vi "VisualizeNHRRGS.vi"() -> ()   [LabVIEW 2018, in "Visualization.lvlib" / "VisualizeAcPwr.lvclass"]
doc: "This VI listens for any measurement data associated with the provided PluginName and displays it to the user for analysis. The display is only suitable for data coming from the NHR Regenerative Grid Simulator Plugin."
uses:
  VisualizeAcPwr.lvclass
  AcPwr/AcPwrShared/clMeasurmentData.ctl
  <vilib>/event_ctls.llb/usereventprio.ctl
  VisualizeBase/VisualizeBase_class/Requests/VisUserEventType.ctl
  <vilib>/Utility/error.llb/Error Cluster From Error Code.vi
  <vilib>/ErrorRing/Error Ring.xnode
  VisualizeBase/VisualizeBase_class/VisualizeBase.lvclass
  <userlib>/NIST/NISTErrorLib/NISTErrorLib.lvlib
  AcPwr/AcPwrShared/AcPwrShared.lvlib
panel:
  out "NHRRGS":waveform(dbl)[](graph)=[{"t0"=timestamp(3657200531.6397257 s since 1904-01-01), "dt"=1.0, "Y"=[46.19]}, {"t0"=timestamp(3657200531.6397257 s since 1904-01-01), "dt"=1.0, "Y"=[2.0]}, {"t0"=timestamp(3657200531.6397257 s since 1904-01-01), "dt"=1.0, "Y"=[60.0]}]
  out "Status Byte Register":T1(array[cluster])
  out "Incorrect DataType?":bool
  in  "PluginName":string="AcPwr.NHRRGS0"
  in  "PlotYAxis":u32[](array[numeric])=[0, 1, 0] max=1
  out "ErrorArray":errorcluster[](array[cluster])
  in  "btnStop":bool
  in  "btnReset":bool
  in  "btnClear":bool
  # "0=Left Axis and 1=Right Axis"
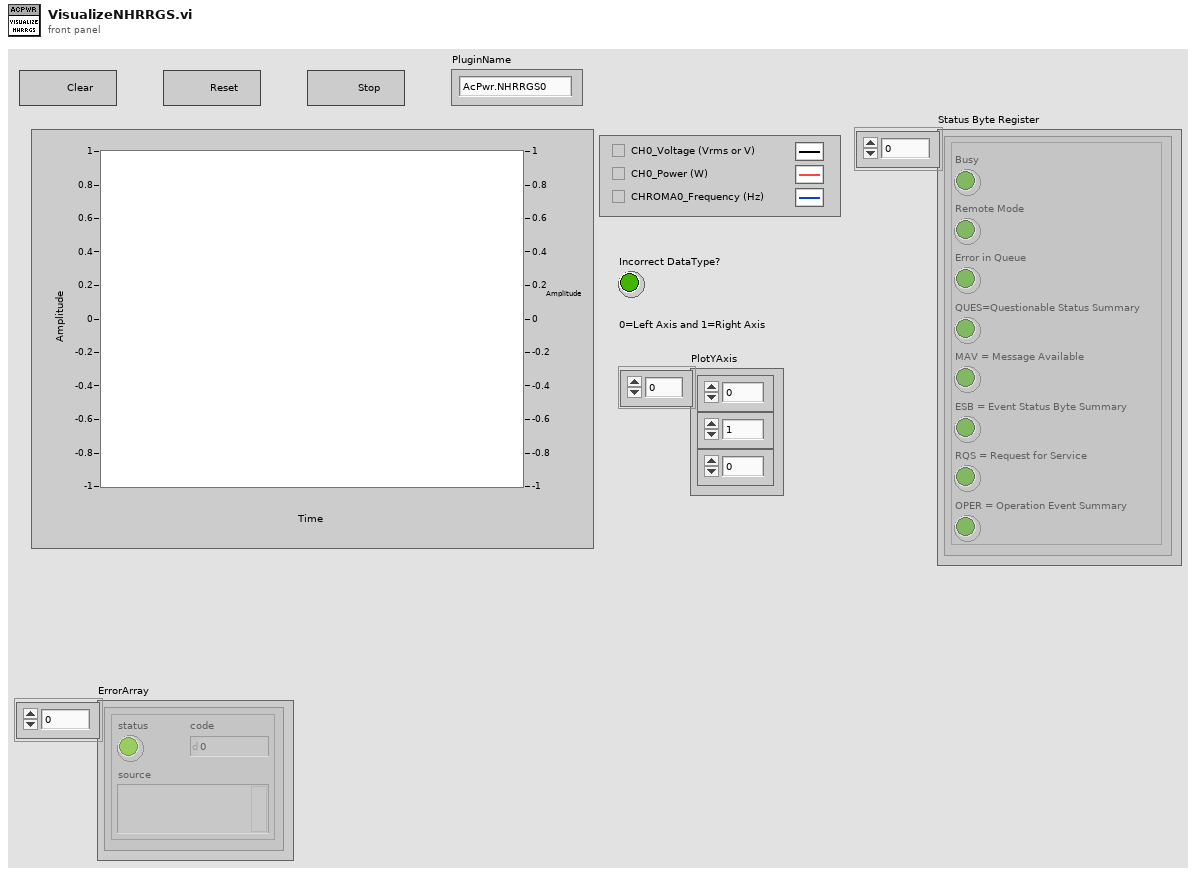
[diagram p1: front panel]
types:
  T1 = cluster{"Busy":bool, "Remote Mode":bool, "Error in Queue":bool, "QUES=Questionable Status Summary":bool, "MAV = Message Available":bool, "ESB = Event Status Byte Summary":bool, "RQS = Request for Service":bool, "OPER = Operation Event Summary":bool}[]
  T2 = typedef "Visualization.lvlib/VisualizeBase.lvclass/VisRequestEvents.ctl" = cluster{"StopRequest":refnum<user-event>, "ResetRequest":refnum<user-event>, "FP Pop In or Out":refnum<user-event>}
  T3 = typedef "AcPwrShared.lvlib/AcPwrBroadcastEvents.ctl" = cluster{"DidInit":refnum<user-event>, "StatusUpdate":refnum<user-event>, "ErrorReport":refnum<user-event>, "DidStop":refnum<user-event>, "PathToINI":refnum<user-event>, "Measurements":refnum<user-event>, "LoadConfigFile":refnum<user-event>, "GetSettings":refnum<user-event>, "SetSettings":refnum<user-event>, "GetType&ID":refnum<user-event>, "GotSettings":refnum<user-event>}
  T4 = typedef "AcPwrShared.lvlib/clMeasurmentData.ctl" = cluster{"MeasName":string, "XML Data":string, "WaveformData":waveform(dbl)[]}
  T5 = typedef "Visualization.lvlib/VisualizeBase.lvclass/VisUserEventType.ctl" = cluster{"BusIndex":i8, "Data":variant}
  T6 = typedef "usereventprio.ctl" = enum32{"high priority", "normal priority"}
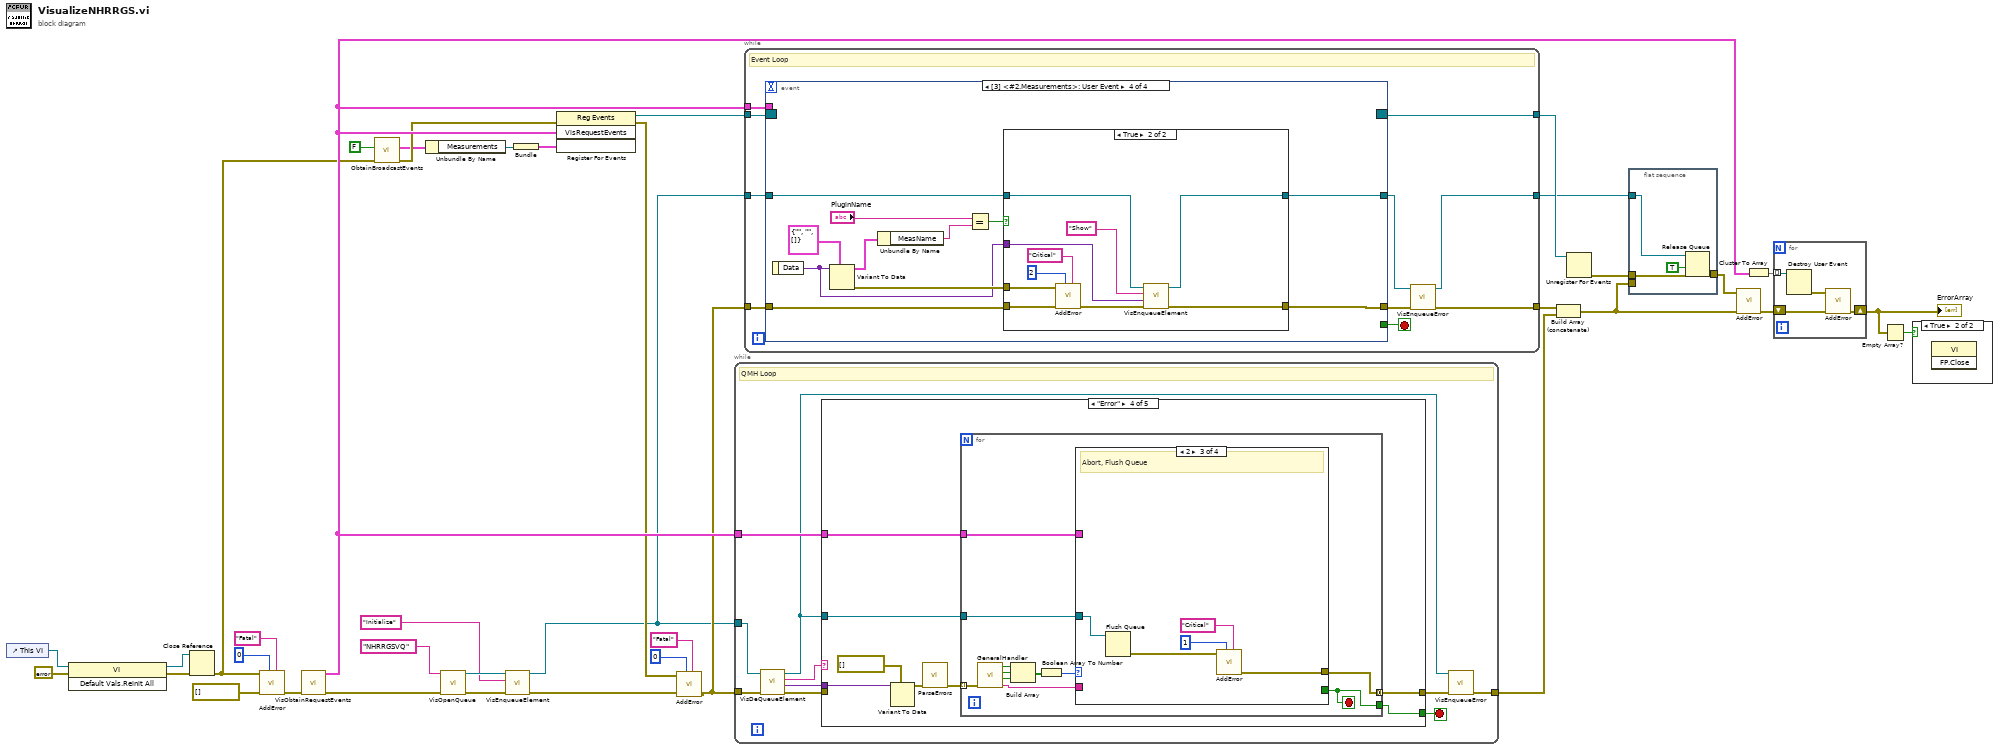
[diagram p0: block diagram]
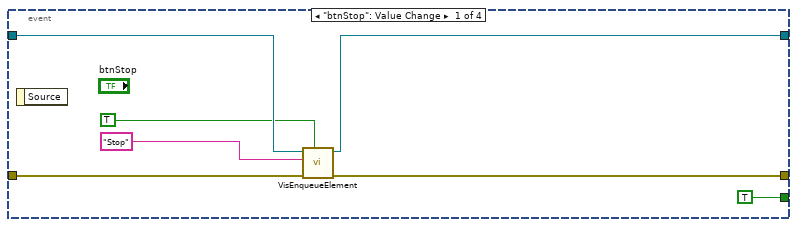
[diagram p2: hidden frame]
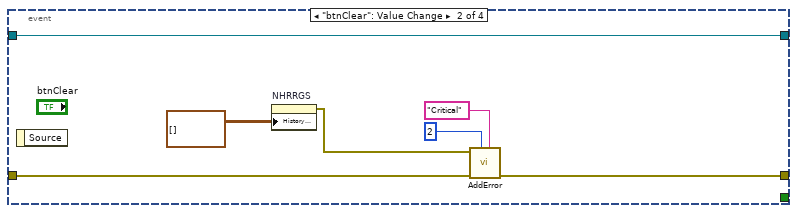
[diagram p3: hidden frame]
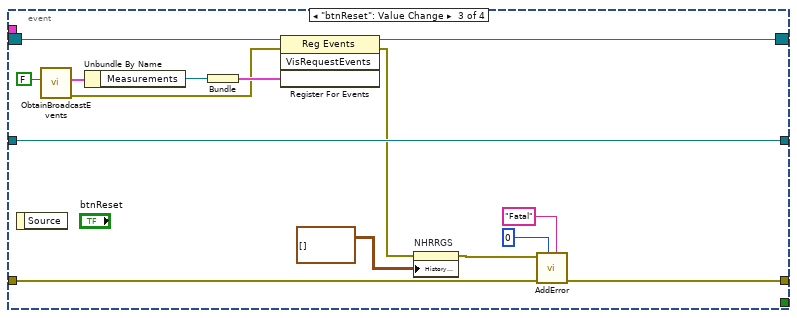
[diagram p4: hidden frame]
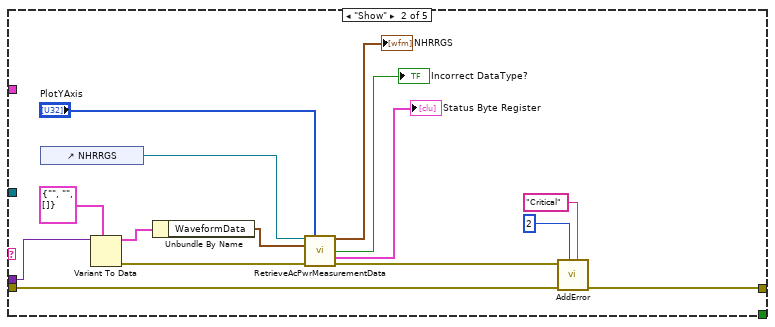
[diagram p7: hidden frame]
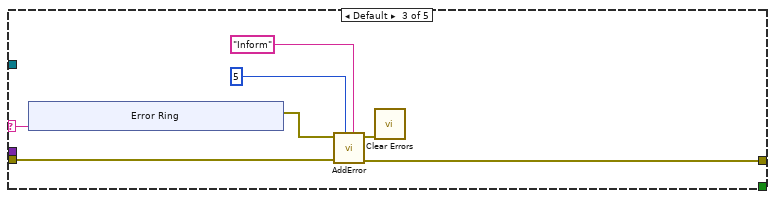
[diagram p8: hidden frame]
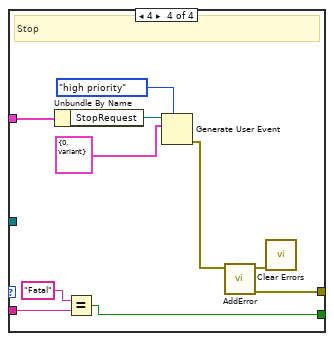
[diagram p11: hidden frame]
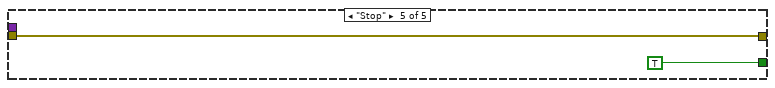
[diagram p12: hidden frame]
diagram:
  n1 = control-ref of="This VI"() -> (w25:refnum<vi>)
  n2 = invoke class="VI" method="Default Vals.Reinit All"(reference=w25, error in=errorcluster {"status"=FALSE, "code"=0, "source"=""} ("error in (no error)")) -> (reference out=w22:refnum<vi>, error out=w23:errorcluster)  [unwired: 1 in, 1 out]
  n3 = Close Reference(reference=w22, error in (no error)=w23) -> (error out=w13:errorcluster)
  n4 = call <userlib>:"AddError.vi"("Severity"="Fatal" ("String"), "Priority"=u8 0, "ErrorArray In"=errorcluster[] [] ("ErrorArray"), "error in (no error)"=w13) -> ("ErrorArray Out"=w37:errorcluster[])  [unwired: 6 in, 1 out]
  n5 = call "VisObtainRequestEvents.vi"("Error"=w37) -> ("Error"=w5:errorcluster[], "VisRequestEvents"=w29:T2)  [unwired: 9 in]
  n6 = call "ObtainBroadcastEvents.vi"("error in (no error)"=w13, "CreateNew? (F)"=FALSE) -> ("error out"=w11:errorcluster, "clAcPwrEvents"=w10:T3)  [unwired: 8 in]
  n7 = Unbundle By Name(w10) -> ("Measurements"=w27:refnum<user-event>)
  n8 = call "VisOpenQueue.vi"("Error Array In"=w5, "QueueName"="NHRRGSVQ" ("QueuName")) -> ("Error Array Out"=w8:errorcluster[], "queue out"=w7:refnum<queue>)  [unwired: 8 in]
  n9 = call "VisEnqueueElement.vi"("Error Array In"=w8, "Message"="Initialize", "queue in"=w7) -> ("Error Array Out"=w4:errorcluster[], "queue out"=w1:refnum<queue>)  [unwired: 7 in]
  n10 = Bundle("Measurements"=w27) -> (w26:cluster{"Measurements":refnum<user-event>})  [unwired: 1 in]
  n11 = register-events(error in=w11, w29, w26) -> (reference out=w38:refnum<event-registration>, error out=w2:errorcluster)  [unwired: 1 in]
  n12 = call <userlib>:"AddError.vi"("Severity"="Fatal" ("String"), "Priority"=u8 0, "ErrorArray In"=w4, "error in (no error)"=w2) -> ("ErrorArray Out"=w3:errorcluster[])  [unwired: 6 in, 1 out]
  n13 = while {
    tunnel: w3 -> [w46]
    tunnel: [w41] -> w33
    tunnel: w29 -> [w47]
    tunnel: w1 -> [w42]
    stop <- w48 stop-if-true
    # "QMH Loop"
    n14 = call "VisDeQueueElement.vi"("Error Array In"=w46, "Queue In"=w42) -> ("Error Array Out"=w45:errorcluster[], "Data"=w44:variant, "Message"=w43:string, "Queue Out"=w39:refnum<queue>)  [unwired: 6 in]
    n15 = case shown="\"Error\"" w43 {
      selector: w43 -> [_ _ w71 _ _]
      tunnel: w44 -> [_ w56 _ w86 _]
      tunnel: w45 -> [w49 w61 w69 _ w113]
      tunnel: [w49 w64 w68 w82 w113] -> w40
      tunnel: [_ _ _ w81 TRUE] -> w48
      tunnel: w47 -> [_ _ _ w80 _]
      tunnel: w39 -> [_ _ _ w79 _]
      frame "Initialize" {
      }
      frame "Show" {
        n16 = control-ref of="NHRRGS"() -> (w58:refnum<vi>)
        n17 = Variant To Data(type=T4 {"MeasName"="", "XML Data"="", "WaveformData"=[]} ("MeasurmentDataCluster"), Variant=w56) -> (data=w54:T4, error out=w55:errorcluster)  [unwired: 1 in]
        n18 = Unbundle By Name(w54) -> ("WaveformData"=w51:waveform(dbl)[])
        n19 = call "RetrieveAcPwrMeasurementData.vi"("WaveformChartReference"=w58, "PlotYScale"="PlotYAxis", "WaveformArrayIn"=w51, "error in (no error)"=w55) -> ("WaveformArrayOut"=→"NHRRGS":waveform(dbl)[], "Incorrect DataType?"=→"Incorrect DataType?":bool, "Status Byte Register(NHRRGS)"=→"Status Byte Register":T1, "error out"=w52:errorcluster)  [unwired: 7 in, 1 out]
        n20 = call <userlib>:"AddError.vi"("Severity"="Critical" ("String"), "Priority"=u8 2, "ErrorArray In"=w61, "error in (no error)"=w52) -> ("ErrorArray Out"=w64:errorcluster[])  [unwired: 6 in, 1 out]
      }
      frame Default {
        n21 = xnode "Error Ring"("parameter 0"=w71) -> ("error out"=w70:errorcluster)
        n22 = call <userlib>:"AddError.vi"("Severity"="Inform" ("String"), "Priority"=u8 5, "ErrorArray In"=w69, "error in (no error)"=w70) -> ("ErrorArray Out"=w68:errorcluster[], "error out"=w67:errorcluster)  [unwired: 6 in]
        n23 = call <vilib>:"Clear Errors.vi"("error in (no error)"=w67) -> ()  [unwired: 5 in, 2 out]
      }
      frame "Error" {
        n24 = Variant To Data(type=errorcluster[] [], Variant=w86) -> (data=w84:errorcluster[])  [unwired: 1 in, 1 out]
        n25 = call <userlib>:"ParseErrors.vi"("ErrorArray"=w84) -> ("ErrorArray"=w83:errorcluster[])  [unwired: 8 in, 2 out]
        n26 = for {
          tunnel: w83 -> [w97] mode=indexing
          tunnel: [w91] -> w82 mode=concatenating
          tunnel: [w89] -> w81
          tunnel: w80 -> [w88]
          tunnel: w79 -> [w87]
          stop <- w89 stop-if-true
          n27 = call <userlib>:"GeneralHandler.vi"("error in (no error)"=w97) -> ("Severity"=w90:string, "Stop"=w94:bool, "Abort"=w95:bool, "Continue"=w96:bool)  [unwired: 6 in, 1 out]
          n28 = Build Array(w96, w95, w94) -> (w93:bool[])
          n29 = Boolean Array To Number(Boolean array=w93) -> (number=w92:u32)
          n30 = case shown="2" w92 {
            tunnel: [_ _ w102 w111] -> w91
            tunnel: w90 -> [_ _ _ w106]
            tunnel: [_ _ _ w104] -> w89
            tunnel: w88 -> [_ _ _ w103]
            tunnel: w87 -> [_ _ w98 _]
            frame 0, Default {
              # "No Dialog"
            }
            frame 1 {
              # "Continue"
            }
            frame 2 {
              # "Abort, Flush Queue"
              n31 = Flush Queue(queue=w98) -> (error out=w101:errorcluster)  [unwired: 1 in, 2 out]
              n32 = call <userlib>:"AddError.vi"("Severity"="Critical" ("String"), "Priority"=u8 1, "error in (no error)"=w101) -> ("ErrorArray Out"=w102:errorcluster[])  [unwired: 7 in, 1 out]
            }
            frame 4 {
              # "Stop"
              n33 = Unbundle By Name(w103) -> ("StopRequest"=w112:refnum<user-event>)
              n34 = Equal?(x="Fatal", y=w106) -> (x = y?=w104:bool)
              n35 = Generate User Event(priority (normal)=usereventprio."high priority", user event=w112, event data cluster=T5 {"BusIndex"=0, "Data"=variant} ("event data")) -> (error out=w110:errorcluster)  [unwired: 1 in, 1 out]
              n36 = call <userlib>:"AddError.vi"("error in (no error)"=w110) -> ("ErrorArray Out"=w111:errorcluster[], "error out"=w107:errorcluster)  [unwired: 9 in]
              n37 = call <vilib>:"Clear Errors.vi"("error in (no error)"=w107) -> ()  [unwired: 5 in, 2 out]
            }
          }
        }
      }
      frame "Stop" {
      }
    }
    n38 = call "VisEnqueueError.vi"("Error Array In"=w40, "Queue in"=w39) -> ("Error Array Out"=w41:errorcluster[])  [unwired: 8 in, 1 out]
  }
  n39 = while {
    tunnel: w38 -> [w124]
    tunnel: [w117] -> w34
    tunnel: [w122] -> w36
    tunnel: w29 -> [w121]
    tunnel: w3 -> [w120]
    tunnel: w1 -> [w119]
    tunnel: [w115] -> w20
    stop <- w123 stop-if-true
    # "Event Loop"
    n40 = event shown="[3] <#2.Measurements>: User Event" {
      selector: w124 -> [_ _ w153 _]
      dyn-events: [_ _ w152 _] -> w122
      timeout: _ -> [_ _ _ _]
      tunnel: [TRUE _ _ _] -> w123
      tunnel: [w129 w135 w146 w164] -> w118
      tunnel: w121 -> [_ _ _ _]
      tunnel: w120 -> [w130 w134 w145 w160]
      tunnel: w119 -> [w128 w138 w147 w162]
      tunnel: [w127 w138 w147 w161] -> w116
      event "btnStop": Value Change {
        n41 = event-data() -> ()  [unwired: 1 in, 1 out]
        n42 = call "VisEnqueueElement.vi"("Priority? (F)"=TRUE, "Error Array In"=w130, "Message"="Stop", "queue in"=w128) -> ("Error Array Out"=w129:errorcluster[], "queue out"=w127:refnum<queue>)  [unwired: 6 in]
      }
      event "btnClear": Value Change {
        n43 = event-data() -> ()  [unwired: 1 in, 1 out]
        n44 = property on="NHRRGS" class="WFChart (strict)"("History Data"=waveform(dbl)[][] [] ("NHRRGS")) -> (error out=w132:errorcluster)  [unwired: 2 in, 1 out]
        n45 = call <userlib>:"AddError.vi"("Severity"="Critical" ("String"), "Priority"=u8 2, "ErrorArray In"=w134, "error in (no error)"=w132) -> ("ErrorArray Out"=w135:errorcluster[])  [unwired: 6 in, 1 out]
      }
      event "btnReset": Value Change {
        n46 = event-data() -> ()  [unwired: 1 in, 1 out]
        n47 = call "ObtainBroadcastEvents.vi"("CreateNew? (F)"=FALSE) -> ("error out"=w148:errorcluster, "clAcPwrEvents"=w149:T3)  [unwired: 9 in]
        n48 = Unbundle By Name(w149) -> ("Measurements"=w151:refnum<user-event>)
        n49 = Bundle("Measurements"=w151) -> (w150:cluster{"Measurements":refnum<user-event>})  [unwired: 1 in]
        n50 = register-events(reference=w153, error in=w148, w150) -> (reference out=w152:refnum<event-registration>, error out=w142:errorcluster)  [unwired: 1 in]
        n51 = property on="NHRRGS" class="WFChart (strict)"(error in=w142, "History Data"=waveform(dbl)[][] [] ("NHRRGS")) -> (error out=w141:errorcluster)  [unwired: 1 in, 1 out]
        n52 = call <userlib>:"AddError.vi"("Severity"="Fatal" ("String"), "Priority"=u8 0, "ErrorArray In"=w145, "error in (no error)"=w141) -> ("ErrorArray Out"=w146:errorcluster[])  [unwired: 6 in, 1 out]
      }
      event User Event {
        n53 = event-data() -> ("Data"=w154:variant)  [unwired: 1 in]
        n54 = Variant To Data(type=T4 {"MeasName"="", "XML Data"="", "WaveformData"=[]} ("MeasurmentDataCluster"), Variant=w154) -> (data=w157:T4, error out=w159:errorcluster)  [unwired: 1 in]
        n55 = Unbundle By Name(w157) -> ("MeasName"=w155:string)
        n56 = Equal?(x="PluginName", y=w155) -> (x = y?=w156:bool)
        n57 = case shown="True" w156 {
          tunnel: w154 -> [_ w168]
          tunnel: [w166 w171] -> w164
          tunnel: w160 -> [w166 w173]
          tunnel: w162 -> [w165 w169]
          tunnel: [w165 w170] -> w161
          tunnel: w159 -> [_ w172]
          frame False {
          }
          frame True {
            n58 = call <userlib>:"AddError.vi"("Severity"="Critical" ("String"), "Priority"=u8 2, "ErrorArray In"=w173, "error in (no error)"=w172) -> ("ErrorArray Out"=w174:errorcluster[])  [unwired: 6 in, 1 out]
            n59 = call "VisEnqueueElement.vi"("Error Array In"=w174, "Data"=w168, "Message"="Show", "queue in"=w169) -> ("Error Array Out"=w171:errorcluster[], "queue out"=w170:refnum<queue>)  [unwired: 6 in]
          }
        }
      }
    }
    n60 = call "VisEnqueueError.vi"("Error Array In"=w118, "Queue in"=w116) -> ("Error Array Out"=w117:errorcluster[], "Queue out"=w115:refnum<queue>)  [unwired: 8 in]
  }
  n61 = Build Array (concatenate)(w34, w33) -> (w14:errorcluster[])
  n62 = Unregister For Events(event registration refnum=w36) -> (error out=w32:errorcluster)  [unwired: 1 in]
  n63 = flat-sequence {
    tunnel: w32 -> [w178]
    tunnel: [w180] -> w31
    tunnel: w20 -> [w179]
    tunnel: w14 -> [_]
    frame #0 {
      n64 = Release Queue(queue=w179, force destroy? (F)=TRUE, error in (no error)=w178) -> (error out=w180:errorcluster)  [unwired: 2 out]
    }
  }
  n65 = call <userlib>:"AddError.vi"("ErrorArray In"=w14, "error in (no error)"=w31) -> ("ErrorArray Out"=w30:errorcluster[])  [unwired: 8 in, 1 out]
  n66 = Cluster To Array(cluster=w29) -> (array=w35:refnum<user-event>[])
  n67 = for {
    tunnel: w35 -> [w184] mode=indexing
    shift-right: [w183] -> w21
    shift-left: w30 -> [w182]
    n68 = Destroy User Event(user event=w184) -> (error out=w181:errorcluster)  [unwired: 1 in]
    n69 = call <userlib>:"AddError.vi"("ErrorArray In"=w182, "error in (no error)"=w181) -> ("ErrorArray Out"=w183:errorcluster[])  [unwired: 8 in, 1 out]
  }
  "ErrorArray" <- w21
  n70 = Empty Array?(array=w21) -> (empty?=w28:bool)
  n71 = case shown="True" w28 {
    frame False {
    }
    frame True {
      n72 = invoke class="VI" method="FP.Close"() -> ()  [unwired: 3 in, 3 out]
    }
  }
